vi "Machines - Create New Machine (SubVI).vi"(8 "error in":errorcluster) -> (0 "error out":errorcluster, 5 "close?":bool)   [LabVIEW 2019]
uses:
  Controls/Machine name-state.ctl
  Controls/FGV States.ctl
panel:
  in  "Max Load":dbl
  in  "Displacement":u16(ring) caption="Displacement Transducer" items=["Not Assigned", "Motor 1", "Motor 2", "LC 1", "LC 2", "LC 3"]
  in  "Transducer":u16(ring) caption="Load/Pressure Transducer" items=["Not Assigned", "LC 1", "LC 2", "LC 3"]
  in  "Motor Control":u16(ring) items=["Not Assigned", "Motor 1", "Motor 2"]
  in  "OK":bool
  in  "Give a name for the machine":string
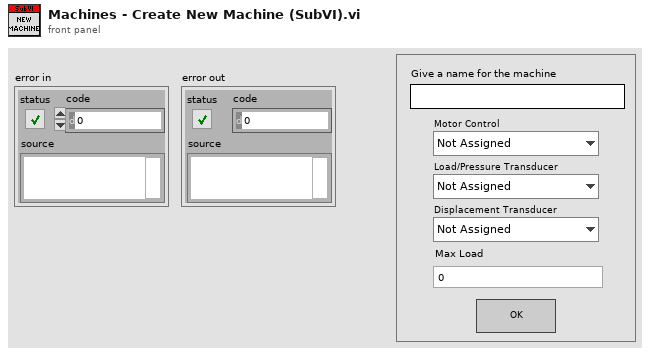
[diagram p1: front panel]
types:
  T1 = typedef "Machine name-state.ctl" = enum16{"Init", "Idle", "Insert", "Update", "Close"}
  T2 = typedef "FGV States.ctl" = enum16{"Read", "Write"}
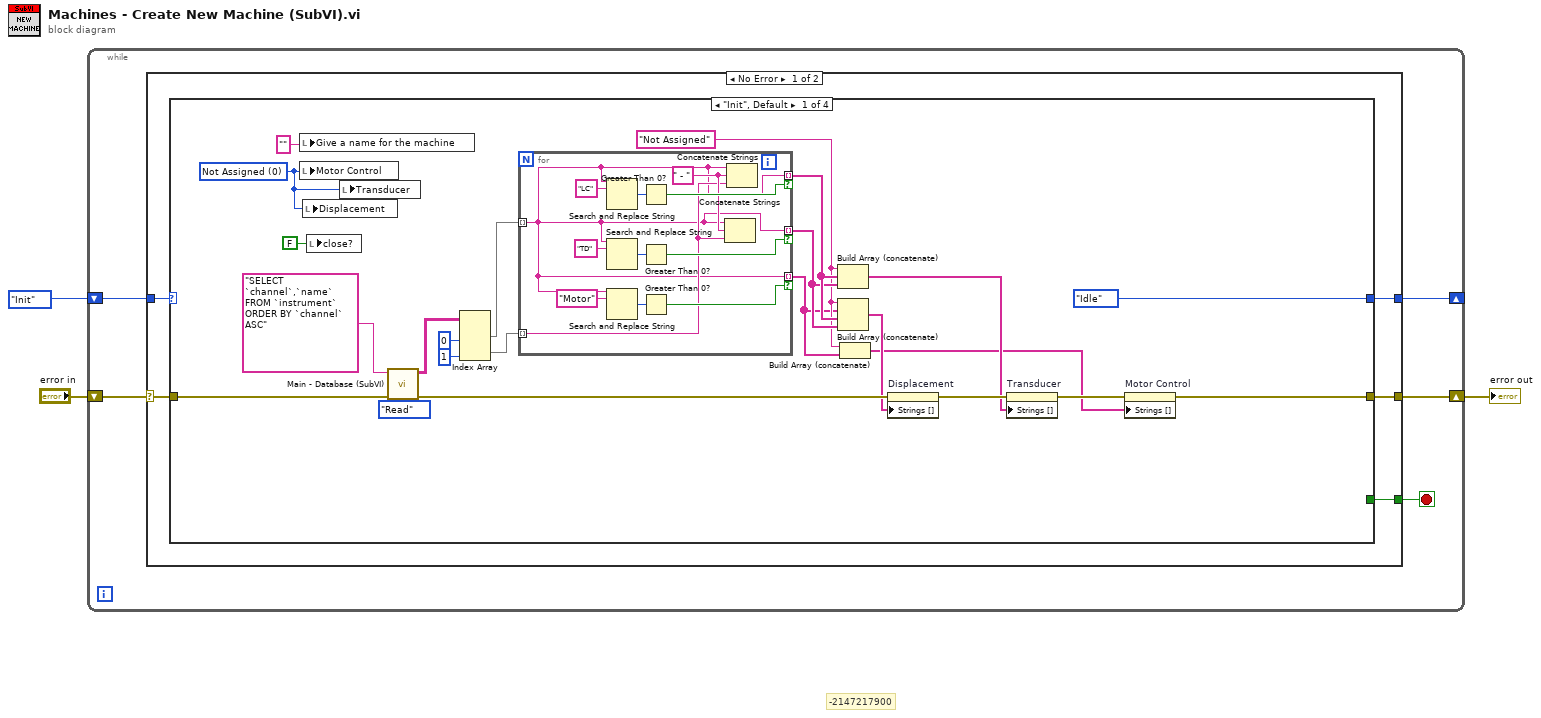
[diagram p0: block diagram]
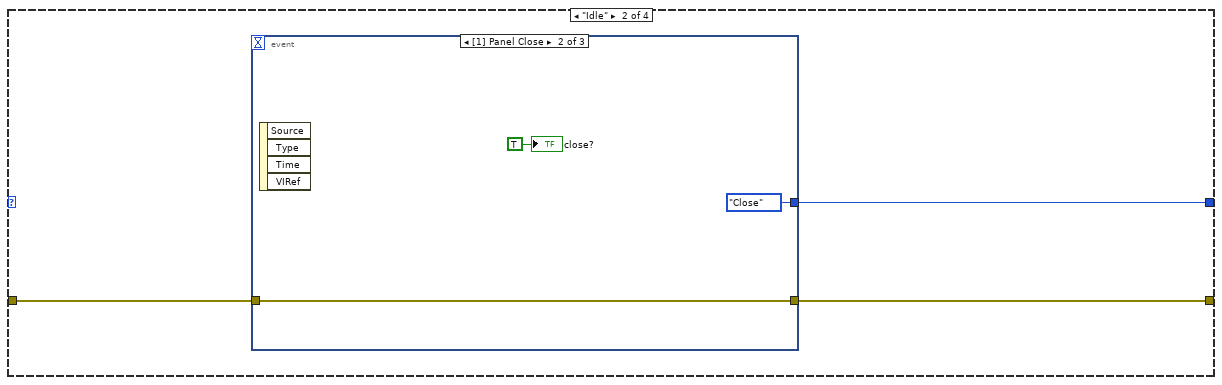
[diagram p2: hidden frame]
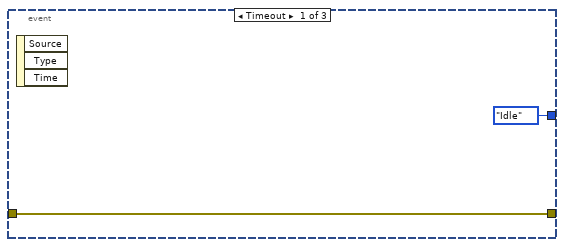
[diagram p3: hidden frame]
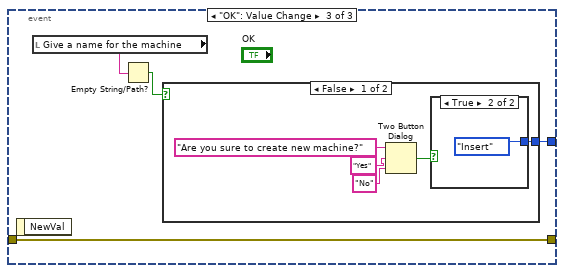
[diagram p4: hidden frame]
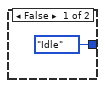
[diagram p5: hidden frame]
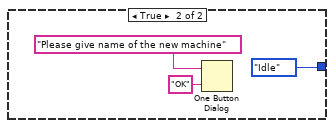
[diagram p6: hidden frame]
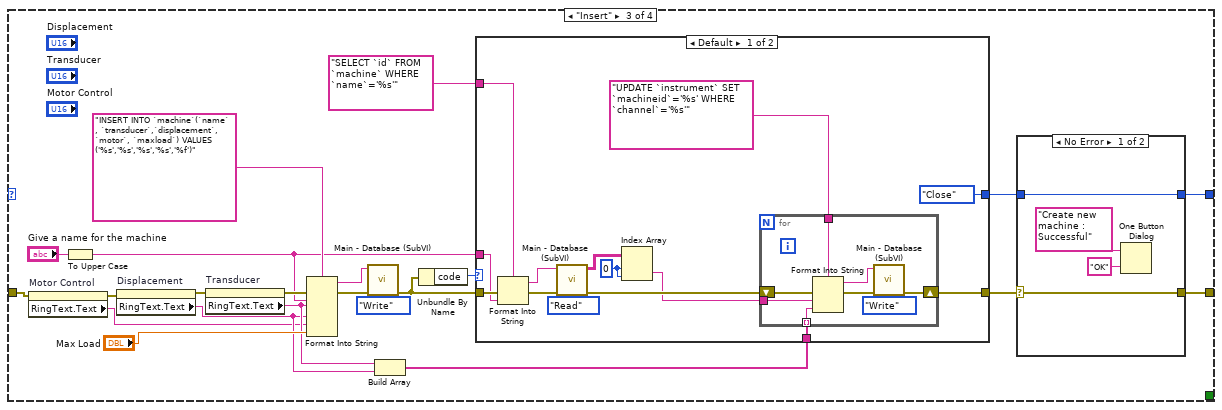
[diagram p7: hidden frame]
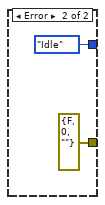
[diagram p8: hidden frame]
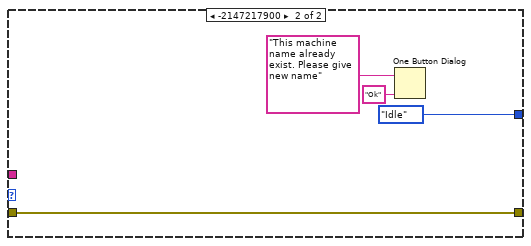
[diagram p9: hidden frame]
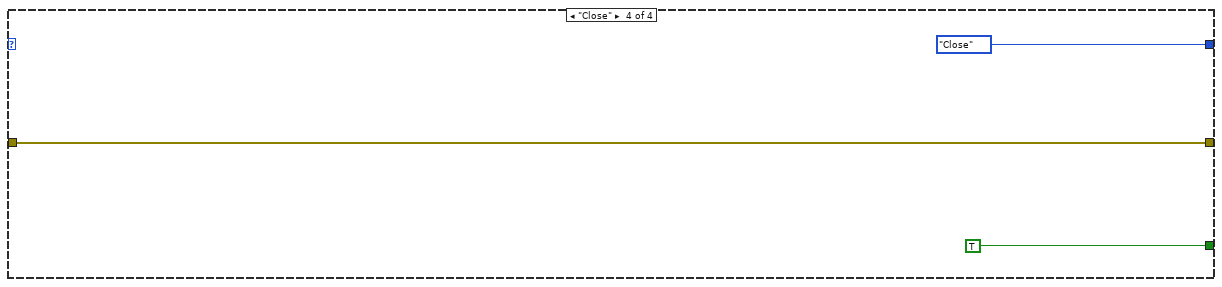
[diagram p10: hidden frame]
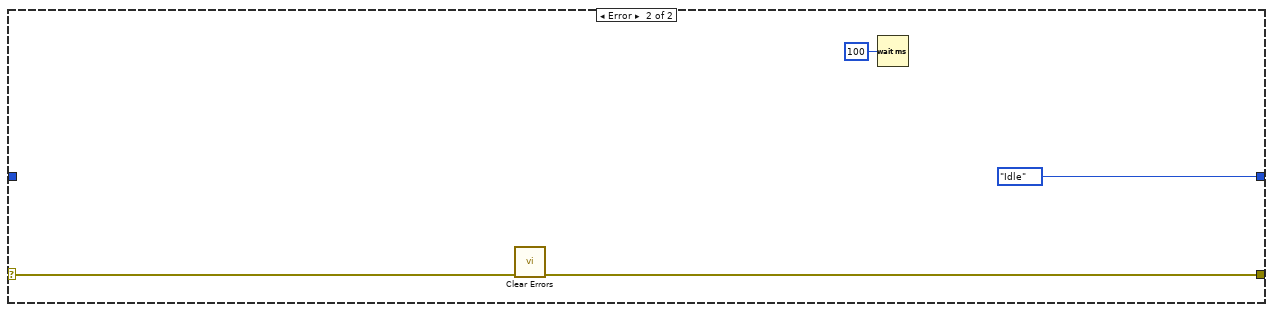
[diagram p11: hidden frame]
diagram:
  # "-2147217900"
  n1 = while {
    shift-right: [w7] -> w2
    shift-left: "error in" -> [w8]
    shift-right: [w5] -> _
    shift-left: Machine_name-state."Init" -> [w6]
    stop <- w4 stop-if-true
    n2 = case shown="No Error" w8 {
      selector: w8 -> [w13 w131]
      tunnel: [w12 w130] -> w7
      tunnel: w6 -> [w11 _]
      tunnel: [w10 Machine_name-state."Idle"] -> w5
      tunnel: [w9 _] -> w4
      frame No Error {
        n3 = case shown="\"Init\", Default" w11 {
          tunnel: w13 -> [w27 w51 w88 w127]
          tunnel: [w17 w50 w71 w127] -> w12
          tunnel: [Machine_name-state."Idle" w49 w73 Machine_name-state."Close"] -> w10
          tunnel: [_ _ _ TRUE] -> w9
          frame "Init", Default {
            w23 = u16 0 items=["Not Assigned", "Motor 1", "Motor 2", "Motor 3", "Motor 4", "Motor 5", "Motor 6", "Motor 7", "Motor 8", "Motor 9"] ("Motor Control")
            w16 = "Not Assigned"
            n4 = local write "Give a name for the machine"("" ("Give a name for the station")) -> ()
            n5 = local write "Motor Control"(w23) -> ()
            n6 = local write "Displacement"(w23) -> ()
            n7 = local write "close?"(FALSE ("close?")) -> ()
            n8 = local write "Transducer"(w23) -> ()
            n9 = call "Main - Database (SubVI).vi"("Enum"=FGV_States."Read", "error in (no error)"=w27, "SQL query"="SELECT `channel`,`name` FROM `instrument` ORDER BY `channel` ASC") -> ("error out"=w26:errorcluster, "data"=w32:string[][])  [unwired: 7 in]
            n10 = Index Array(array=w32, index (col) #1=0 ("disabled index (col)"), index (col) #2=1 ("index (col)")) -> (element #1=w30:string[], element #2=w20:string[])  [unwired: 2 in]
            n11 = for {
              tunnel: w30 -> [w37] mode=indexing
              tunnel: [w37] -> w15 mode=indexing if=w46
              tunnel: [w37] -> w28 mode=indexing if=w41
              tunnel: [w37] -> w29 mode=indexing if=w40
              tunnel: w20 -> [w38] mode=indexing
              w39 = " - " ("string")
              n12 = Search and Replace String(input string=w37, search string="LC") -> (number of replacements=w42:i32)  [unwired: 6 in, 3 out]
              n13 = Search and Replace String(input string=w37, search string="TD") -> (number of replacements=w45:i32)  [unwired: 6 in, 3 out]
              n14 = Search and Replace String(input string=w37, search string="Motor") -> (number of replacements=w47:i32)  [unwired: 6 in, 3 out]
              n15 = Greater Than 0?(x=w42) -> (x > 0?=w40:bool)
              n16 = Greater Than 0?(x=w45) -> (x > 0?=w41:bool)
              n17 = Greater Than 0?(x=w47) -> (x > 0?=w46:bool)
              n18 = Concatenate Strings(w37, w39, w38) -> ()  [unwired: 1 out]
              n19 = Concatenate Strings(w37, w39, w38) -> ()  [unwired: 1 out]
            }
            n20 = Build Array (concatenate)(w16, w29, w28) -> (w24:string[])
            n21 = Build Array (concatenate)(w16, w15, w29, w28) -> (w25:string[])
            n22 = Build Array (concatenate)(w16, w15) -> (w14:string[])
            n23 = property on="Displacement" class="Ring (strict)"(error in=w26, "Strings []"=w25) -> (error out=w35:errorcluster)  [unwired: 1 in, 1 out]
            n24 = property on="Transducer" class="Ring (strict)"(error in=w35, "Strings []"=w24) -> (error out=w18:errorcluster)  [unwired: 1 in, 1 out]
            n25 = property on="Motor Control" class="Ring (strict)"(error in=w18, "Strings []"=w14) -> (error out=w17:errorcluster)  [unwired: 1 in, 1 out]
          }
          frame "Idle" {
            n26 = event shown="[1] Panel Close" {
              selector: _ -> [_ _ _]
              dyn-events: _ -> [_ _ _]
              timeout: _ -> [_ _ _]
              tunnel: w51 -> [w53 w56 w60]
              tunnel: [w53 w56 w60] -> w50
              tunnel: [Machine_name-state."Idle" Machine_name-state."Close" w59] -> w49
              event Timeout {
                n27 = event-data() -> ()  [unwired: 1 in, 3 out]
              }
              event Panel Close {
                n28 = event-data() -> ()  [unwired: 1 in, 4 out]
                "close?" <- TRUE ("close?")
              }
              event "OK": Value Change {
                n29 = event-data() -> ()  [unwired: 1 in, 1 out]
                n30 = local read "Give a name for the machine"() -> (w58:string)
                n31 = Empty String/Path?(string/path=w58) -> (empty?=w57:bool)
                n32 = case shown="False" w57 {
                  tunnel: [w65 Machine_name-state."Idle"] -> w59
                  frame False {
                    n33 = Two Button Dialog(message="Are you sure to create new machine?", 1:"No" ("F button name (\"Cancel\")"), 2:"Yes" ("T button name (\"OK\")")) -> (T button?=w61:bool)
                    n34 = case shown="True" w61 {
                      tunnel: [Machine_name-state."Idle" Machine_name-state."Insert"] -> w65
                      frame False {
                      }
                      frame True {
                      }
                    }
                  }
                  frame True {
                    n35 = One Button Dialog(message="Please give name of the new machine", button name ("OK")="OK") -> ()  [unwired: 1 out]
                  }
                }
              }
            }
          }
          frame "Insert" {
            n36 = property on="Motor Control" class="Ring (strict)"(error in=w88) -> (error out=w90:errorcluster, "RingText.Text"=w76:string)  [unwired: 1 in, 1 out]
            n37 = To Upper Case(1:"Give a name for the machine") -> (0:w80:string)
            n38 = property on="Displacement" class="Ring (strict)"(error in=w90) -> (error out=w89:errorcluster, "RingText.Text"=w77:string)  [unwired: 1 in, 1 out]
            n39 = property on="Transducer" class="Ring (strict)"(error in=w89) -> (error out=w83:errorcluster, "RingText.Text"=w78:string)  [unwired: 1 in, 1 out]
            n40 = Format Into String(format string="INSERT INTO `machine`(`name` , `transducer`,`displacement`, `motor`, `maxload`) VALUES ('%s','%s','%s','%s','%f')" ("SQL query"), error in=w83, w80, w78, w77, w76, "Max Load") -> (resulting string=w87:string, error out=w86:errorcluster)  [unwired: 1 in]
            n41 = call "Main - Database (SubVI).vi"("Enum"=FGV_States."Write", "error in (no error)"=w86, "SQL query"=w87) -> ("error out"=w82:errorcluster)  [unwired: 7 in, 1 out]
            n42 = Build Array(w78, w77) -> (w75:string[])
            n43 = Unbundle By Name(w82) -> ("code"=w91:i32)
            n44 = case shown="Default" w91 {
              tunnel: [Machine_name-state."Close" Machine_name-state."Idle"] -> w72
              tunnel: [w111 w121] -> w74
              tunnel: w82 -> [w108 w121]
              tunnel: w80 -> [w105 _]
              tunnel: "SELECT `id` FROM `machine` WHERE `name`='%s'" ("message") -> [w107 _]
              tunnel: w75 -> [w99 _]
              frame Default {
                w103 = 0 ("index (row)")
                n45 = Format Into String(format string=w107, error in=w108, w105) -> (resulting string=w106:string, error out=w109:errorcluster)  [unwired: 1 in]
                n46 = call "Main - Database (SubVI).vi"("Enum"=FGV_States."Read", "error in (no error)"=w109, "SQL query"=w106) -> ("error out"=w102:errorcluster, "data"=w104:string[][])  [unwired: 7 in]
                n47 = Index Array(array=w104, index (row)=w103, index (col)=w103) -> (element=w100:string)
                n48 = for {
                  tunnel: "UPDATE `instrument` SET `machineid`='%s' WHERE `channel`='%s'" ("message") -> [w115]
                  tunnel: w100 -> [w114]
                  shift-right: [w119] -> w111
                  shift-left: w102 -> [w118]
                  tunnel: w99 -> [w113] mode=indexing
                  n49 = Format Into String(format string=w115, error in=w118, w114, w113) -> (resulting string=w116:string, error out=w117:errorcluster)  [unwired: 1 in]
                  n50 = call "Main - Database (SubVI).vi"("Enum"=FGV_States."Write", "error in (no error)"=w117, "SQL query"=w116) -> ("error out"=w119:errorcluster)  [unwired: 7 in, 1 out]
                }
              }
              frame -2147217900 {
                n51 = One Button Dialog(message="This machine name already exist. Please give new name", button name ("OK")="Ok") -> ()  [unwired: 1 out]
              }
            }
            n52 = case shown="No Error" w74 {
              selector: w74 -> [w93 _]
              tunnel: [w94 Machine_name-state."Idle"] -> w73
              tunnel: w72 -> [w94 _]
              tunnel: [w93 errorcluster {"status"=FALSE, "code"=0, "source"=""} ("error IO")] -> w71
              frame No Error {
                n53 = One Button Dialog(message="Create new machine : Successful", button name ("OK")="OK") -> ()  [unwired: 1 out]
              }
              frame Error {
              }
            }
          }
          frame "Close" {
          }
        }
      }
      frame Error {
        n54 = call <vilib>:"Clear Errors.vi"("error in (no error)"=w131) -> ("error out"=w130:errorcluster)  [unwired: 5 in, 1 out]
        n55 = Wait (ms)(milliseconds to wait=u32 100) -> ()  [unwired: 1 out]
      }
    }
  }
  "error out" <- w2
